vi "Standard PLC Byte Stream to G Object.vi"(8 "error in (no error)":errorcluster, 9 "PLC Type":T1, 10 "Byte Stream":u8[](array[numeric]), 11 "TwinCAT ADS in":refnum<class "TwinCAT ADS.lvclass">) -> (0 "error out":errorcluster, 2 "Value":variant, 3 "TwinCAT ADS out":refnum<class "TwinCAT ADS.lvclass">)   [LabVIEW 2018, in "TwinCAT ADS.lvclass"]
uses:
  TwinCAT ADS.lvclass
  Controls/PLC Type.ctl
  9a8c356b-cf55-4838-9201-0532b80217b2.vi
  06482052-d1f9-4f29-aca9-908031c6a69f.vi
  b9242781-96b0-446e-9150-452b1084ed54.vi
  5fbe6976-0b86-40a2-b7b6-3748894f0071.vi
  c4de1741-fffd-4fed-ba25-d7b4acbf0555.vi
  20356124-05d2-4a04-a5d1-e69adc4c58c2.vi
  67ddb754-0fbe-43d9-9e61-34d6659124ef.vi
  e3d41cb3-d20e-45e9-8252-e41884a8f4d0.vi
  46ba2a54-cc07-4222-9a0e-bd972edfcef0.vi
  6b416cf7-30dc-48a3-9278-9d800f443678.vi
  5857d013-9824-4299-a2d7-53efdc0d26c5.vi
  006b0e7e-7e80-41f3-be4e-1f3da8479fae.vi
  28d9c90b-5f2a-4c58-95e2-5fc46303b0fd.vi
  99b7bc4a-962e-4818-aa5d-444f23f83b11.vi
  8b7c42c8-9170-4542-8f35-15cbeddc22cb.vi
  65a091fa-0bd2-4a35-ae2b-3fa5e90d1994.vi
  4b7d3a7d-7f1b-46f0-9357-48cb72148c56.vi
  b431183c-2ad5-4c6d-9bfa-a53b18913682.vi
  30c6c28a-53c3-4e33-80b1-b22f521e1f67.vi
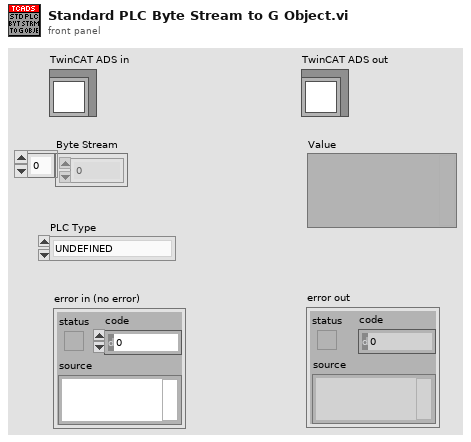
[diagram p1: front panel]
types:
  T1 = typedef "TwinCAT ADS.lvclass/PLC Type.ctl" = enum16{"UNDEFINED", "INT", "DINT", "REAL", "LREAL", "SINT", "BYTE", "UINT", "UDINT", "LINT", "ULINT", "STRING", "WSTRING", "BOOL", "TIME", "LTIME", "DATE", "DT", "TOD", "ARRAY", "JAGGED ARRAY", "STRUCT", "FUNCTION BLOCK", "POINTER", "USER DEFINED"}
  T2 = typedef "LVDateTimeRec.ctl" = cluster{"fractional second":dbl, "second":i32, "minute":i32, "hour":i32, "day of month":i32, "month":i32, "year":i32, "day of week":i32, "day of year":i32, "DST":i32}
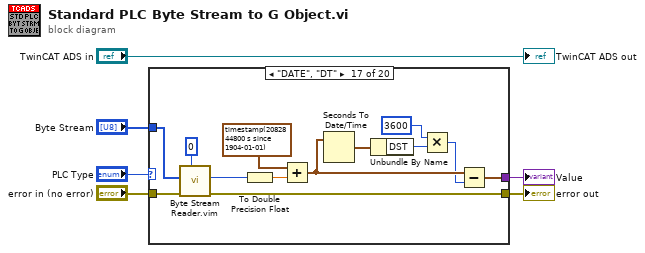
[diagram p0: block diagram]
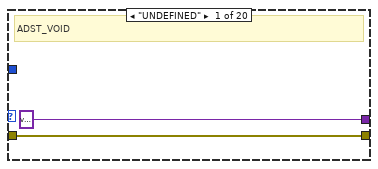
[diagram p2: hidden frame]
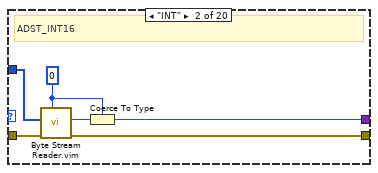
[diagram p3: hidden frame]
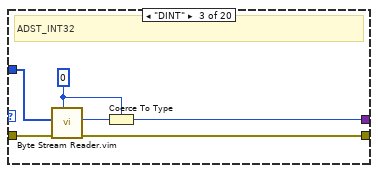
[diagram p4: hidden frame]
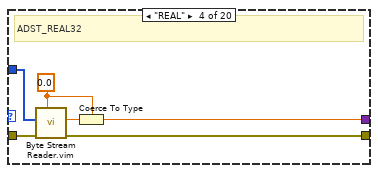
[diagram p5: hidden frame]
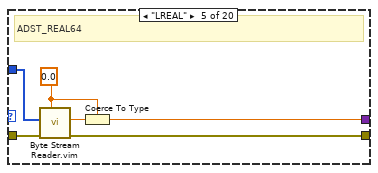
[diagram p6: hidden frame]
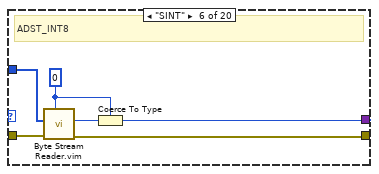
[diagram p7: hidden frame]
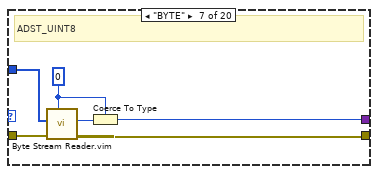
[diagram p8: hidden frame]
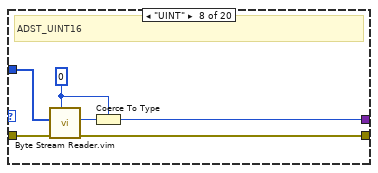
[diagram p9: hidden frame]
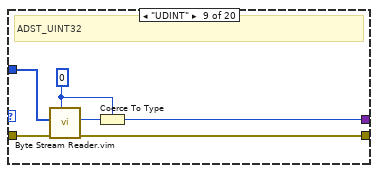
[diagram p10: hidden frame]
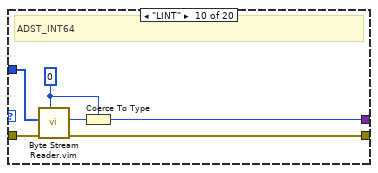
[diagram p11: hidden frame]
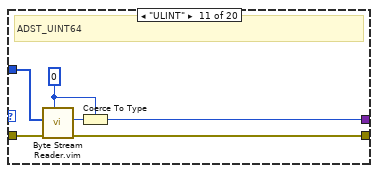
[diagram p12: hidden frame]
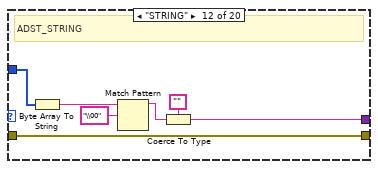
[diagram p13: hidden frame]
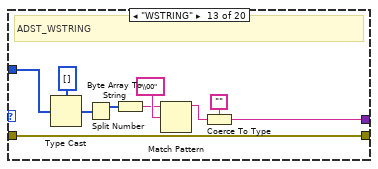
[diagram p14: hidden frame]
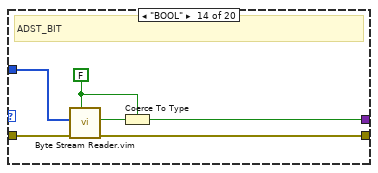
[diagram p15: hidden frame]
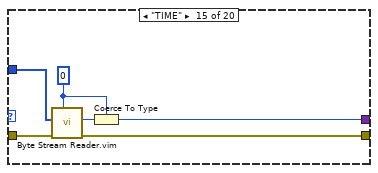
[diagram p16: hidden frame]
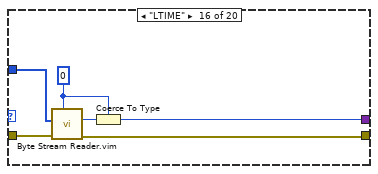
[diagram p17: hidden frame]
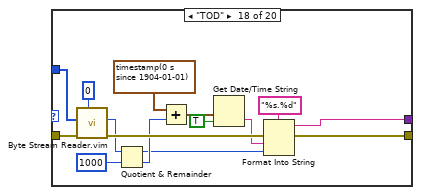
[diagram p18: hidden frame]
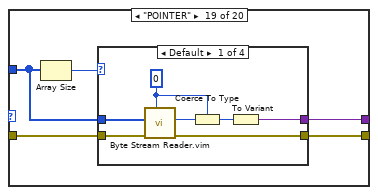
[diagram p19: hidden frame]
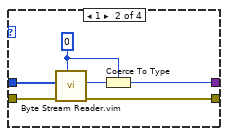
[diagram p20: hidden frame]
diagram:
  n1 = case shown="\"DATE\", \"DT\"" "PLC Type" {
    tunnel: [variant w9 w15 w21 w27 w33 w39 w45 w51 w57 w63 w69 w76 w86 w93 w98 w104 w122 w133 w162] -> w4
    tunnel: "error in (no error)" -> [w7 w14 w20 w26 w32 w38 w44 w50 w56 w62 w68 w72 w79 w91 w97 w103 w115 w130 w136 w163]
    tunnel: [w7 w13 w19 w25 w31 w37 w43 w49 w54 w60 w66 w72 w79 w89 w95 w101 w112 w120 w132 w163] -> w3
    tunnel: "Byte Stream" -> [_ w12 w18 w24 w30 w36 w42 w48 w55 w61 w67 w75 w84 w90 w96 w102 w114 w128 w134 w162]
    frame "UNDEFINED" {
      # "ADST_VOID"
    }
    frame "INT" {
      w10 = i16 0
      # "ADST_INT16"
      n2 = call "Byte Stream Reader.vim"("Type"=w10, "error in (no error)"=w14, "Byte Stream"=w12) -> ("error out"=w13:errorcluster, "Value"=w11:i16)  [unwired: 7 in]
      n3 = Coerce To Type(0:w11, 1:w10) -> (2:w9:i16)
    }
    frame "DINT" {
      w16 = 0
      # "ADST_INT32"
      n4 = call "Byte Stream Reader.vim"("Type"=w16, "error in (no error)"=w20, "Byte Stream"=w18) -> ("error out"=w19:errorcluster, "Value"=w17:i32)  [unwired: 7 in]
      n5 = Coerce To Type(0:w17, 1:w16) -> (2:w15:i32)
    }
    frame "REAL" {
      w22 = sgl 0.0
      # "ADST_REAL32"
      n6 = call "Byte Stream Reader.vim"("Type"=w22, "error in (no error)"=w26, "Byte Stream"=w24) -> ("error out"=w25:errorcluster, "Value"=w23:sgl)  [unwired: 7 in]
      n7 = Coerce To Type(0:w23, 1:w22) -> (2:w21:sgl)
    }
    frame "LREAL" {
      w28 = 0.0
      # "ADST_REAL64"
      n8 = call "Byte Stream Reader.vim"("Type"=w28, "error in (no error)"=w32, "Byte Stream"=w30) -> ("error out"=w31:errorcluster, "Value"=w29:dbl)  [unwired: 7 in]
      n9 = Coerce To Type(0:w29, 1:w28) -> (2:w27:dbl)
    }
    frame "SINT" {
      w34 = i8 0
      # "ADST_INT8"
      n10 = call "Byte Stream Reader.vim"("Type"=w34, "error in (no error)"=w38, "Byte Stream"=w36) -> ("error out"=w37:errorcluster, "Value"=w35:i8)  [unwired: 7 in]
      n11 = Coerce To Type(0:w35, 1:w34) -> (2:w33:i8)
    }
    frame "BYTE" {
      w40 = u8 0
      # "ADST_UINT8"
      n12 = call "Byte Stream Reader.vim"("Type"=w40, "error in (no error)"=w44, "Byte Stream"=w42) -> ("error out"=w43:errorcluster, "Value"=w41:u8)  [unwired: 7 in]
      n13 = Coerce To Type(0:w41, 1:w40) -> (2:w39:u8)
    }
    frame "UINT" {
      w46 = u16 0
      # "ADST_UINT16"
      n14 = call "Byte Stream Reader.vim"("Type"=w46, "error in (no error)"=w50, "Byte Stream"=w48) -> ("error out"=w49:errorcluster, "Value"=w47:u16)  [unwired: 7 in]
      n15 = Coerce To Type(0:w47, 1:w46) -> (2:w45:u16)
    }
    frame "UDINT" {
      w52 = u32 0
      # "ADST_UINT32"
      n16 = call "Byte Stream Reader.vim"("Type"=w52, "error in (no error)"=w56, "Byte Stream"=w55) -> ("error out"=w54:errorcluster, "Value"=w53:u32)  [unwired: 7 in]
      n17 = Coerce To Type(0:w53, 1:w52) -> (2:w51:u32)
    }
    frame "LINT" {
      w58 = i64 0
      # "ADST_INT64"
      n18 = call "Byte Stream Reader.vim"("Type"=w58, "error in (no error)"=w62, "Byte Stream"=w61) -> ("error out"=w60:errorcluster, "Value"=w59:i64)  [unwired: 7 in]
      n19 = Coerce To Type(0:w59, 1:w58) -> (2:w57:i64)
    }
    frame "ULINT" {
      w65 = u64 0
      # "ADST_UINT64"
      n20 = call "Byte Stream Reader.vim"("Type"=w65, "error in (no error)"=w68, "Byte Stream"=w67) -> ("error out"=w66:errorcluster, "Value"=w64:u64)  [unwired: 7 in]
      n21 = Coerce To Type(0:w64, 1:w65) -> (2:w63:u64)
    }
    frame "STRING" {
      # "ADST_STRING"
      n22 = Byte Array To String(unsigned byte array=w75) -> (string=w74:string)
      n23 = Match Pattern(string=w74, regular expression="\\00") -> (before substring=w70:string)  [unwired: 1 in, 3 out]
      n24 = Coerce To Type(0:w70, 1:"") -> (2:w69:string)
    }
    frame "WSTRING" {
      # "ADST_WSTRING"
      n25 = Type Cast(type=u16[] [] ("Byte Stream"), x=w84) -> (*(type *) &x=w80:u16[])
      n26 = Split Number(x=w80) -> (hi(x)=w81:u8[])  [unwired: 1 out]
      n27 = Byte Array To String(unsigned byte array=w81) -> (string=w82:string)
      n28 = Match Pattern(string=w82, regular expression="\\00") -> (before substring=w77:string)  [unwired: 1 in, 3 out]
      n29 = Coerce To Type(0:w77, 1:"") -> (2:w76:string)
    }
    frame "BOOL" {
      w87 = FALSE
      # "ADST_BIT"
      n30 = call "Byte Stream Reader.vim"("Type"=w87, "error in (no error)"=w91, "Byte Stream"=w90) -> ("error out"=w89:errorcluster, "Value"=w88:bool)  [unwired: 7 in]
      n31 = Coerce To Type(0:w88, 1:w87) -> (2:w86:bool)
    }
    frame "TIME" {
      w92 = u32 0
      n32 = call "Byte Stream Reader.vim"("Type"=w92, "error in (no error)"=w97, "Byte Stream"=w96) -> ("error out"=w95:errorcluster, "Value"=w94:u32)  [unwired: 7 in]
      n33 = Coerce To Type(0:w94, 1:w92) -> (2:w93:u32)
    }
    frame "LTIME" {
      w99 = u64 0
      n34 = call "Byte Stream Reader.vim"("Type"=w99, "error in (no error)"=w103, "Byte Stream"=w102) -> ("error out"=w101:errorcluster, "Value"=w100:u64)  [unwired: 7 in]
      n35 = Coerce To Type(0:w100, 1:w99) -> (2:w98:u64)
    }
    frame "DATE", "DT" {
      n36 = call "Byte Stream Reader.vim"("Type"=u32 0, "error in (no error)"=w115, "Byte Stream"=w114) -> ("error out"=w112:errorcluster, "Value"=w111:u32)  [unwired: 7 in]
      n37 = To Double Precision Float(number=w111) -> (double precision float=w113:dbl)
      n38 = Add(x=timestamp(2082844800 s since 1904-01-01) ("time stamp"), y=w113) -> (x+y=w109:timestamp)
      n39 = Seconds To Date/Time(time stamp (now)=w109) -> (date time rec=w108:T2)  [unwired: 1 in]
      n40 = Unbundle By Name(w108) -> ("DST"=w107:i32)
      n41 = Multiply(x=3600, y=w107) -> (x*y=w105:i32)
      n42 = Subtract(x=w109, y=w105) -> (x-y=w104:timestamp)
    }
    frame "TOD" {
      n43 = call "Byte Stream Reader.vim"("Type"=u32 0, "error in (no error)"=w130, "Byte Stream"=w128) -> ("error out"=w131:errorcluster, "Value"=w119:u32)  [unwired: 7 in]
      n44 = Quotient & Remainder(x=w119, y=u32 1000) -> (x-y*floor(x/y)=w118:u32, floor(x/y)=w125:u32)
      n45 = Add(x=timestamp(0 s since 1904-01-01), y=w125) -> (x+y=w124:timestamp)
      n46 = Get Date/Time String(seconds (now)=w124, want seconds? (F)=TRUE) -> (time string=w117:string)  [unwired: 1 in, 1 out]
      n47 = Format Into String(format string="%s.%d", error in=w131, w117, w118) -> (resulting string=w122:string, error out=w120:errorcluster)  [unwired: 1 in]
    }
    frame "POINTER" {
      n48 = Array Size(array=w134) -> (size(s)=w135:i32)
      n49 = case shown="Default" w135 {
        tunnel: w136 -> [w142 w148 w154 w160]
        tunnel: w134 -> [w140 w146 w152 w158]
        tunnel: [w139 w145 w151 w157] -> w132
        tunnel: [w137 w144 w150 w156] -> w133
        frame Default {
          w141 = u64 0
          n50 = call "Byte Stream Reader.vim"("Type"=w141, "error in (no error)"=w142, "Byte Stream"=w140) -> ("error out"=w139:errorcluster, "Value"=w143:u64)  [unwired: 7 in]
          n51 = Coerce To Type(0:w143, 1:w141) -> (2:w138:u64)
          n52 = To Variant(anything=w138) -> (Variant=w137:variant)
        }
        frame 1 {
          w147 = u64 0
          n53 = call "Byte Stream Reader.vim"("Type"=w147, "error in (no error)"=w148, "Byte Stream"=w146) -> ("error out"=w145:errorcluster, "Value"=w149:u64)  [unwired: 7 in]
          n54 = Coerce To Type(0:w149, 1:w147) -> (2:w144:u64)
        }
        frame 2 {
          w153 = u16 0
          n55 = call "Byte Stream Reader.vim"("Type"=w153, "error in (no error)"=w154, "Byte Stream"=w152) -> ("error out"=w151:errorcluster, "Value"=w155:u16)  [unwired: 7 in]
          n56 = Coerce To Type(0:w155, 1:w153) -> (2:w150:u16)
        }
        frame 4 {
          w159 = u32 0
          n57 = call "Byte Stream Reader.vim"("Type"=w159, "error in (no error)"=w160, "Byte Stream"=w158) -> ("error out"=w157:errorcluster, "Value"=w161:u32)  [unwired: 7 in]
          n58 = Coerce To Type(0:w161, 1:w159) -> (2:w156:u32)
        }
      }
    }
    frame Default {
    }
  }
  "error out" <- w3
  "Value" <- w4
  "TwinCAT ADS out" <- "TwinCAT ADS in"
